vi "Intermediate Binding Test.vi"() -> (0 "error out":errorcluster)   [LabVIEW 2014, in "SQLite3LV Tests.lvlib"]
uses:
  SQLite3LV Tests.lvlib
  SQLite3LV/SQLite3 Class/struct_table_info.ctl
  SQLite3LV/Cursor Class/property binding/bind text.vi
  SQLite3LV/Cursor Class/property binding/bind BLOB.vi
  SQLite3LV/Cursor Class/property binding/bind I32.vi
  SQLite3LV/Cursor Class/property binding/bind I64.vi
  SQLite3LV/Cursor Class/property binding/bind DBL.vi
  SQLite3LV/Cursor Class/property binding/column I32.vi
  SQLite3LV/Cursor Class/property binding/column Text.vi
  SQLite3LV/Cursor Class/property binding/column BLOB.vi
  SQLite3LV/Cursor Class/property binding/column DBL.vi
  SQLite3LV/SQLite3 Class/sqlite3.lvclass
  SQLite3LV/Cursor Class/cursor.lvclass
  SQLite3LV/SQLite3LV.lvlib
panel:
  in  "last name LIKE":string="%"
  out "table info.":T1[](array[typedef])
  out "Table Names":string[](array[string])
  out "Array":T2(array[cluster])
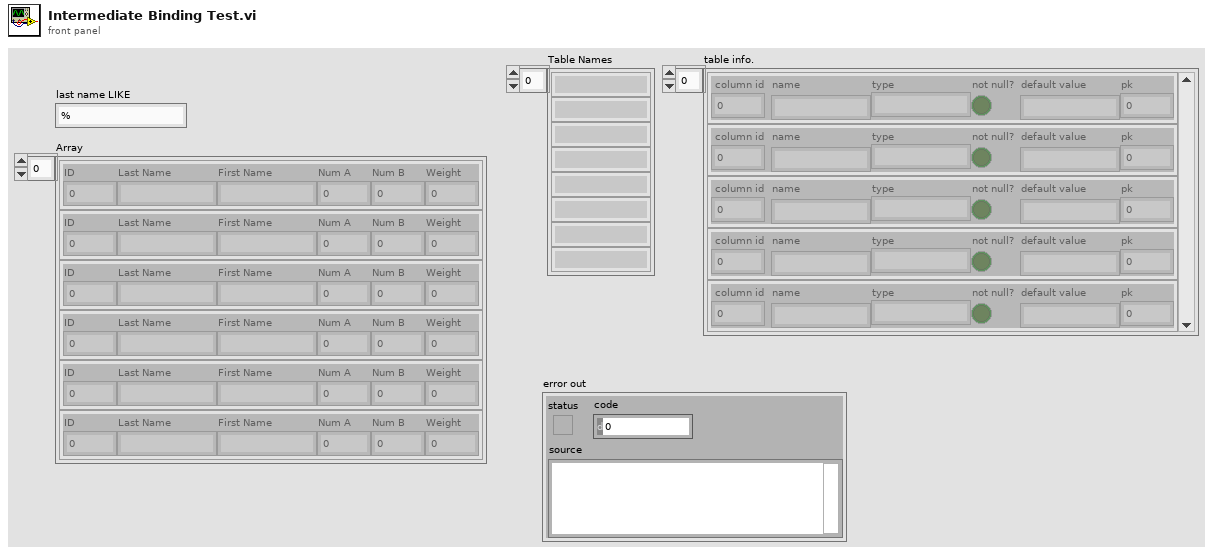
[diagram p1: front panel]
types:
  T1 = typedef "SQLite3LV.lvlib/struct_table_info.ctl" = cluster{" column id":i32, "name":string, "type":string, "not null?":bool, "default value":string, "pk":i32}
  T2 = cluster{"ID":i32, "Last Name":string, "First Name":string, "Num A":i32, "Num B":i32, "Weight":dbl}[]
  T3 = cluster{"property binding:Column I32":i32, "property binding:Column Text":string, "property binding:Column BLOB":string, "property binding:Column I32":i32, "property binding:Column I32":i32, "property binding:Column DBL":dbl}
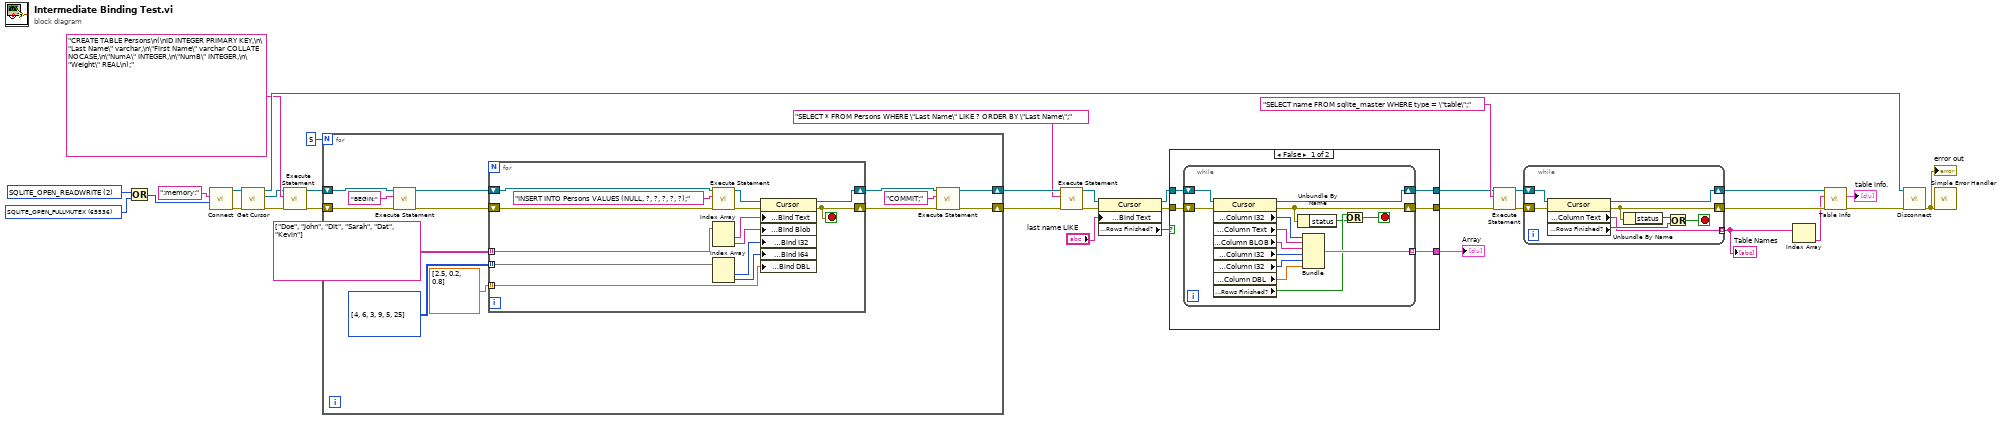
[diagram p0: block diagram]
diagram:
  w34 = u32 65536 items=["SQLITE_OPEN_READONLY"=1, "SQLITE_OPEN_READWRITE"=2, "SQLITE_OPEN_CREATE"=4, "SQLITE_OPEN_DELETEONCLOSE"=8, "SQLITE_OPEN_EXCLUSIVE"=16, "SQLITE_OPEN_AUTOPROXY"=32, "SQLITE_OPEN_URI"=64, "SQLITE_OPEN_MEMORY"=128, "SQLITE_OPEN_MAIN_DB"=256, "SQLITE_OPEN_TEMP_DB"=512, "SQLITE_OPEN_TRANSIENT_DB"=1024, "SQLITE_OPEN_MAIN_JOURNAL"=2048, "SQLITE_OPEN_TEMP_JOURNAL"=4096, "SQLITE_OPEN_SUBJOURNAL"=8192, "SQLITE_OPEN_MASTER_JOURNAL"=16384, "SQLITE_OPEN_NOMUTEX"=32768, "SQLITE_OPEN_FULLMUTEX"=65536, "SQLITE_OPEN_SHAREDCACHE"=131072, "SQLITE_OPEN_PRIVATECACHE"=262144, "SQLITE_OPEN_WAL"=524288] ("SQLITE3 Open Flag")
  w35 = u32 2 items=["SQLITE_OPEN_READONLY"=1, "SQLITE_OPEN_READWRITE"=2, "SQLITE_OPEN_CREATE"=4, "SQLITE_OPEN_DELETEONCLOSE"=8, "SQLITE_OPEN_EXCLUSIVE"=16, "SQLITE_OPEN_AUTOPROXY"=32, "SQLITE_OPEN_URI"=64, "SQLITE_OPEN_MEMORY"=128, "SQLITE_OPEN_MAIN_DB"=256, "SQLITE_OPEN_TEMP_DB"=512, "SQLITE_OPEN_TRANSIENT_DB"=1024, "SQLITE_OPEN_MAIN_JOURNAL"=2048, "SQLITE_OPEN_TEMP_JOURNAL"=4096, "SQLITE_OPEN_SUBJOURNAL"=8192, "SQLITE_OPEN_MASTER_JOURNAL"=16384, "SQLITE_OPEN_NOMUTEX"=32768, "SQLITE_OPEN_FULLMUTEX"=65536, "SQLITE_OPEN_SHAREDCACHE"=131072, "SQLITE_OPEN_PRIVATECACHE"=262144, "SQLITE_OPEN_WAL"=524288] ("SQLITE3 Open Flag")
  n1 = Compound Arithmetic op=OR(w35, w34) -> (w32:u32)
  n2 = call "Connect.vi"("SQLITE3 open flags"=w32, "path"=":memory:" ("path_utf8")) -> ("error out"=w30:errorcluster, "SQLite3LV Connection out"=w31:refnum<class "sqlite3.lvclass">)  [unwired: 8 in]
  n3 = call "Get Cursor.vi"("error in (no error)"=w30, "SQLite3LV Connection in"=w31) -> ("error out"=w13:errorcluster, "SQLite3LV Cursor"=w14:refnum<class "cursor.lvclass">, "SQLite3LV Connection out"=w28:refnum<class "sqlite3.lvclass">)  [unwired: 7 in]
  n4 = call "Execute Statement.vi"("error in (no error)"=w13, "SQL statement"="CREATE TABLE Persons\n(\nID INTEGER PRIMARY KEY,\n\"Last Name\" varchar,\n\"First Name\" varchar COLLATE NOCASE,\n\"NumA\" INTEGER,\n\"NumB\" INTEGER,\n\"Weight\" REAL\n);" ("statement"), "SQLite3LV Cursor in"=w14) -> ("error out"=w25:errorcluster, "SQLite3LV Cursor out"=w26:refnum<class "cursor.lvclass">)  [unwired: 7 in]
  n5 = for {
    N: 5 -> [_]
    shift-right: [w37] -> w24
    shift-left: w26 -> [w46]
    shift-right: [w36] -> w21
    shift-left: w25 -> [w45]
    n6 = call "Execute Statement.vi"("error in (no error)"=w45, "SQL statement"="BEGIN;", "SQLite3LV Cursor in"=w46) -> ("error out"=w42:errorcluster, "SQLite3LV Cursor out"=w43:refnum<class "cursor.lvclass">)  [unwired: 7 in]
    n7 = for {
      shift-right: [w50] -> w40
      shift-left: w43 -> [w62]
      tunnel: string[][] [["Doe", "John"], ["Dit", "Sarah"], ["Dat", "Kevin"]] -> [w58] mode=indexing
      shift-right: [w51] -> w38
      shift-left: w42 -> [w60]
      tunnel: i32[][] [[4, 6], [3, 9], [5, 25]] -> [w56] mode=indexing
      tunnel: dbl[] [2.5, 0.2, 0.8] -> [w53] mode=indexing
      stop <- w51 stop-if-true
      n8 = call "Execute Statement.vi"("error in (no error)"=w60, "SQL statement"="INSERT INTO Persons VALUES (NULL, ?, ?, ?, ?, ?);" ("statement"), "SQLite3LV Cursor in"=w62) -> ("error out"=w52:errorcluster, "SQLite3LV Cursor out"=w59:refnum<class "cursor.lvclass">)  [unwired: 7 in]
      n9 = Index Array(array=w58) -> (element #1=w57:string, element #2=w49:string)  [unwired: 2 in]
      n10 = Index Array(array=w56) -> (element #1=w55:i32, element #2=w54:i32)  [unwired: 2 in]
      n11 = property class="Cursor"(reference=w59, error in=w52, "property binding:Bind Text"=w57, "property binding:Bind Blob"=w49, "property binding:Bind I32"=w55, "property binding:Bind I64"=w54, "property binding:Bind DBL"=w53) -> (reference out=w50:refnum<class "cursor.lvclass">, error out=w51:errorcluster)
    }
    n12 = call "Execute Statement.vi"("error in (no error)"=w38, "SQL statement"="COMMIT;", "SQLite3LV Cursor in"=w40) -> ("error out"=w36:errorcluster, "SQLite3LV Cursor out"=w37:refnum<class "cursor.lvclass">)  [unwired: 7 in]
  }
  n13 = call "Execute Statement.vi"("error in (no error)"=w21, "SQL statement"="SELECT * FROM Persons WHERE \"Last Name\" LIKE ? ORDER BY \"Last Name\";" ("statement"), "SQLite3LV Cursor in"=w24) -> ("error out"=w5:errorcluster, "SQLite3LV Cursor out"=w20:refnum<class "cursor.lvclass">)  [unwired: 7 in]
  n14 = property class="Cursor"(reference=w20, error in=w5, "property binding:Bind Text"="last name LIKE") -> (reference out=w6:refnum<class "cursor.lvclass">, error out=w4:errorcluster, "property binding:Rows Finished?"=w2:bool)
  n15 = case shown="False" w2 {
    tunnel: [w67 _] -> w19
    tunnel: [w66 w82] -> w18
    tunnel: [w65 w83] -> w17
    tunnel: w6 -> [w64 w83]
    tunnel: w4 -> [w63 w82]
    frame False {
      n16 = while {
        shift-right: [w79] -> w65
        shift-left: w64 -> [w81]
        shift-right: [w70] -> w66
        shift-left: w63 -> [w80]
        tunnel: [w72] -> w67 mode=indexing
        stop <- w69 stop-if-true
        n17 = property class="Cursor"(reference=w81, error in=w80) -> (reference out=w79:refnum<class "cursor.lvclass">, error out=w70:errorcluster, "property binding:Column I32"=w78:i32, "property binding:Column Text"=w77:string, "property binding:Column BLOB"=w76:string, "property binding:Column I32"=w75:i32, "property binding:Column I32"=w74:i32, "property binding:Column DBL"=w73:dbl, "property binding:Rows Finished?"=w71:bool)
        n18 = Unbundle By Name(w70) -> ("status"=w68:bool)
        n19 = Bundle("property binding:Column I32"=w78, "property binding:Column Text"=w77, "property binding:Column BLOB"=w76, "property binding:Column I32"=w75, "property binding:Column I32"=w74, "property binding:Column DBL"=w73) -> (w72:T3)  [unwired: 1 in]
        n20 = Or(x=w71, y=w68) -> (x .or. y?=w69:bool)
      }
    }
    frame True {
    }
  }
  "Array" <- w19
  n21 = call "Execute Statement.vi"("error in (no error)"=w18, "SQL statement"="SELECT name FROM sqlite_master WHERE type = \"table\";" ("statement"), "SQLite3LV Cursor in"=w17) -> ("error out"=w15:errorcluster, "SQLite3LV Cursor out"=w16:refnum<class "cursor.lvclass">)  [unwired: 7 in]
  n22 = while {
    shift-right: [w89] -> w12
    shift-left: w16 -> [w91]
    shift-right: [w85] -> w11
    shift-left: w15 -> [w90]
    tunnel: [w87] -> w10 mode=indexing
    stop <- w86 stop-if-true
    n23 = property class="Cursor"(reference=w91, error in=w90) -> (reference out=w89:refnum<class "cursor.lvclass">, error out=w85:errorcluster, "property binding:Column Text"=w87:string, "property binding:Rows Finished?"=w88:bool)
    n24 = Unbundle By Name(w85) -> ("status"=w84:bool)
    n25 = Or(x=w84, y=w88) -> (x .or. y?=w86:bool)
  }
  "Table Names" <- w10
  n26 = Index Array(array=w10) -> (element=w9:string)  [unwired: 1 in]
  n27 = call "Table Info.vi"("error in (no error)"=w11, "table"=w9, "SQLite3LV Cursor in"=w12) -> ("error out"=w8:errorcluster, "table info."=→"table info.":T1[])  [unwired: 6 in, 1 out]
  n28 = call "Disconnect.vi"("error in (no error)"=w8, "SQLite3LV Connection in"=w28) -> ("error out"=w29:errorcluster)  [unwired: 9 in]
  "error out" <- w29
  n29 = call <vilib>:"Simple Error Handler.vi"("error in (no error)"=w29) -> ()  [unwired: 4 in, 5 out]
